vi "Get All Library VIs.vi"(8 "error in":errorcluster, 11 "library ref":refnum<vi>) -> (0 "error out":errorcluster, 3 "vi refs":refnum<vi>[](array[refnum]))   [LabVIEW 2020, in "Build Automation.lvlib"]
uses:
  Build Automation.lvlib
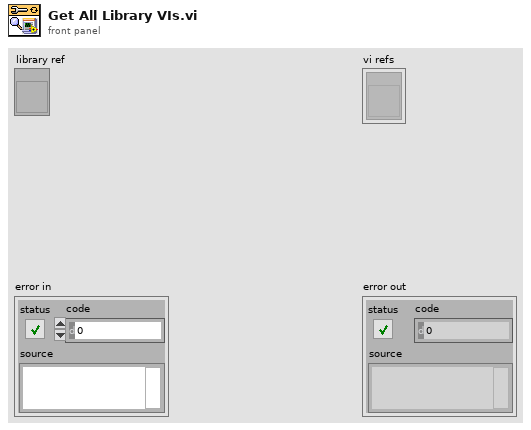
[diagram p1: front panel]
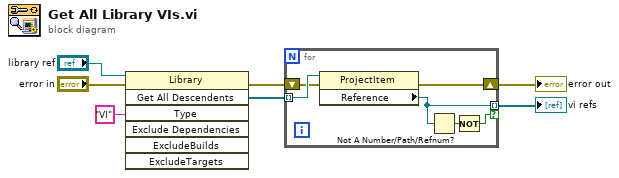
[diagram p0: block diagram]
diagram:
  n1 = invoke class="Library" method="Get All Descendents"(reference="library ref", error in="error in", "Type"="VI") -> (error out=w6:errorcluster, "All Descendents"=w5:refnum<vi>[])  [unwired: 4 in, 5 out]
  n2 = for {
    tunnel: w5 -> [w13] mode=indexing
    shift-right: [w11] -> w3
    shift-left: w6 -> [w12]
    tunnel: [w9] -> w2 mode=indexing if=w8
    n3 = property class="ProjectItem"(reference=w13, error in=w12) -> (error out=w11:errorcluster, "Reference"=w9:refnum<vi>)  [unwired: 1 out]
    n4 = Not A Number/Path/Refnum?(number/path/refnum=w9) -> (NaN/Path/Refnum?=w10:bool)
    n5 = Not(x=w10) -> (.not. x?=w8:bool)
  }
  "error out" <- w3
  "vi refs" <- w2
